vi "MCListbox Event - Add and Remove Buttons.vi"(4 "CellBG New Cells":u32(colorbox)=16777225, 6 "CellBG Unused Cells":u32(colorbox)=16777238, 7 "new element/subarray":string[](array[string]), 8 "Error In":errorcluster, 10 "MCListBox Ref":refnum<vi>[](array[refnum])=[refnum, refnum, refnum], 11 "CtlRef Boolean":refnum<vi>) -> (0 "Error Out":errorcluster)   [LabVIEW 2013]
uses:
  <vilib>/Utility/miscctls.llb/LVRowAndColumnTypeDef.ctl
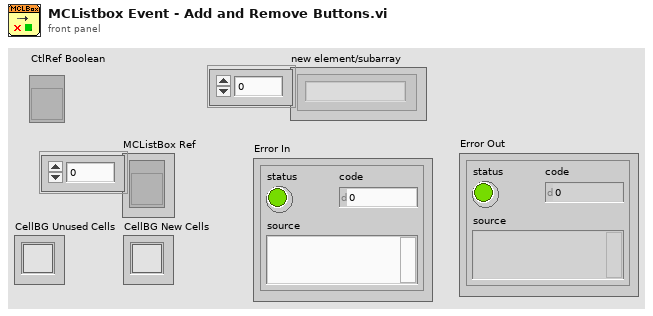
[diagram p1: front panel]
types:
  T1 = typedef "LVRowAndColumnTypeDef.ctl" = cluster{"Row":i32, "Column":i32}
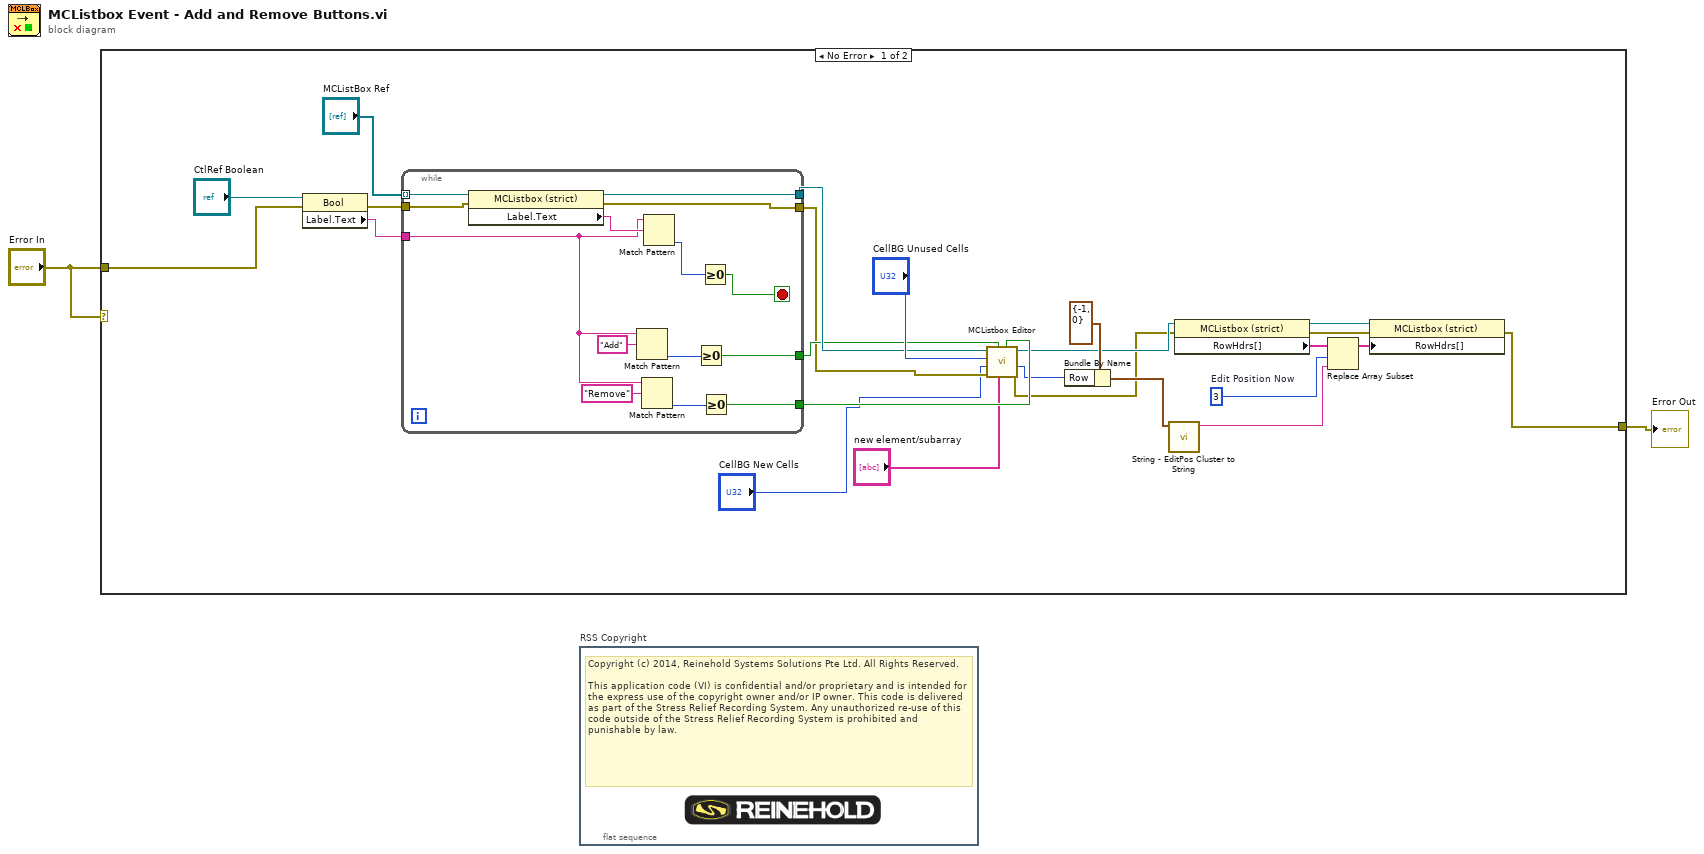
[diagram p0: block diagram]
diagram:
  n1 = case shown="No Error" "Error In" {
    tunnel: "Error In" -> [w17 _]
    tunnel: [w4 _] -> w2
    frame No Error {
      w10 = 3  # Edit Position Now
      n2 = property class="Bool"(reference="CtlRef Boolean", error in=w17) -> (error out=w15:errorcluster, "Label.Text"=w21:string)  [unwired: 1 out]
      n3 = while {
        tunnel: w21 -> [w31]
        tunnel: [w39] -> w24
        tunnel: [w34] -> w23
        tunnel: [w30] -> w22
        tunnel: "MCListBox Ref" -> [w29] mode=indexing
        tunnel: [w28] -> w16
        tunnel: w15 -> [w27]
        stop <- w37 stop-if-true
        n4 = property class="MCListbox (strict)"(reference=w29, error in=w27) -> (reference out=w39:refnum<vi>, error out=w28:errorcluster, "Label.Text"=w40:string)
        n5 = Match Pattern(string=w31, regular expression="Add") -> (offset past match=w35:i32)  [unwired: 1 in, 3 out]
        n6 = Match Pattern(string=w31, regular expression="Remove") -> (offset past match=w33:i32)  [unwired: 1 in, 3 out]
        n7 = Match Pattern(string=w31, regular expression=w40) -> (offset past match=w38:i32)  [unwired: 1 in, 3 out]
        n8 = Greater Or Equal To 0?(x=w35) -> (x >= 0?=w34:bool)
        n9 = Greater Or Equal To 0?(x=w38) -> (x >= 0?=w37:bool)
        n10 = Greater Or Equal To 0?(x=w33) -> (x >= 0?=w30:bool)
      }
      n11 = call "MCListbox Editor.vi"("Remove Row"=w22, "new element/subarray"="new element/subarray", "Add Row Above"=w23, "Error In"=w16, "CellBG New Cells"="CellBG New Cells", "CellBG Unused Cells"="CellBG Unused Cells", "MulticolumnListbox in"=w24) -> ("Error Out"=w6:errorcluster, "Value"=w19:i32, "MulticolumnListbox out"=w13:refnum<vi>)  [unwired: 2 in]
      n12 = Bundle By Name(cluster=T1 {"Row"=-1, "Column"=0} ("Edit Position Now"), "Row"=w19) -> (w8:T1)
      n13 = call "String - EditPos Cluster to String.vi"("EditPos"=w8) -> ("result string"=w7:string)  [unwired: 10 in]
      n14 = property class="MCListbox (strict)"(reference=w13, error in=w6) -> (reference out=w12:refnum<vi>, error out=w5:errorcluster, "RowHdrs[]"=w11:string[])
      n15 = Replace Array Subset(array=w11, new element=w7, index=w10) -> (w9:string[])
      n16 = property class="MCListbox (strict)"(reference=w12, error in=w5, "RowHdrs[]"=w9) -> (error out=w4:errorcluster)  [unwired: 1 out]
    }
    frame Error {
    }
  }
  "Error Out" <- w2
  n17 = flat-sequence "RSS Copyright" {
    frame #0 {
      # "Copyright (c) 2014, Reinehold Systems Solutions Pte Ltd. All Rights Reserved.\n\nThis application code (VI) is confidential and/or proprietary and is intended for the express use of the copyright owner and/or IP owner. This code is delivered as part of the Stress Relief Recording System. Any unauthorized re-use of this code outside of the Stress Relief Recording System is prohibited and punishable by law."
    }
  }
